vi "IDE_Example_Milan.vi"() -> ()   [LabVIEW 2020]
uses:
  Console XCtrl/Console_Xctrl.xctl
  Server XCtrl/Server.xctl
  ColorText/Code.xctl
panel:
  in  "Clean":bool
  in  "PC Save":bool
  in  "Selection":bool
  in  "PC path":path
  in  "Files":bool
  in  "Server":bool
  in  "Help":bool
  in  "Server":path(xcontrol)=path "/Users/crogers/GitHub/Summer2020/LabVIEWCode/Servers/Jens.vi"
  out "REPL":string(xcontrol)
  in  "Clear":bool
  in  "Save":bool
  in  "Stop":bool
  in  "Run":bool
  in  "Name":string="code.py"
  in  "Code":string(xcontrol)="import os\n\nfor i in range(10):\n     print(i)\n"
  # "¨Processor"
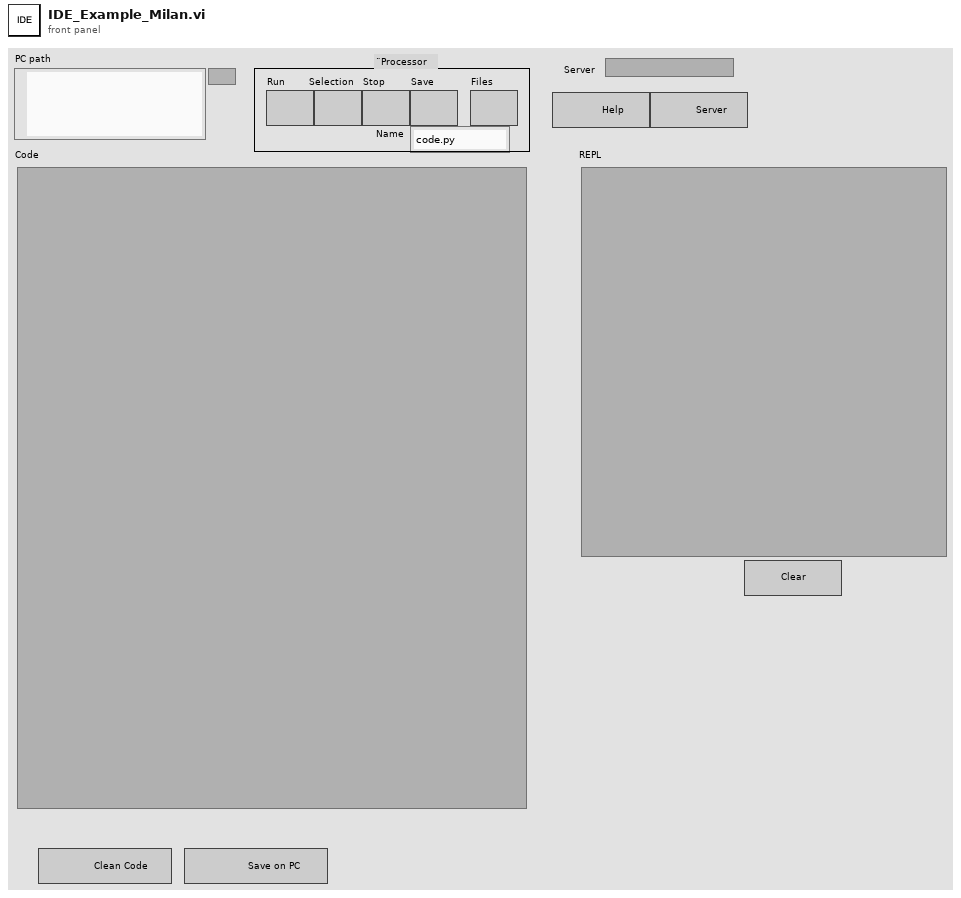
[diagram p1: front panel]
types:
  T1 = cluster{"Quote":u32, "Comment":u32, "Python":u32, "Text":u32, "Triple Quote":u32, "function":u32}
  T2 = enum8{"Enabled", "Disabled", "Disabled and Grayed Out"}
  T3 = typedef "eventvkey.ctl" = enum16{"ASCII", "Enter", "Return", "Shift", "Ctrl", "Alt", "Cmd", "Opt", "Caps", "NumLock", "Clear", "Break", "Up", "Down", "Left", "Right", "Insert", "Delete", "Home", "End", "PageUp", "PageDown", "Escape", "Help", "Pause", "ScrollLock", "F1", "F2", "F3", "F4", "F5", "F6", "F7", "F8", "F9", "F10", "F11", "F12", "F13", "F14", "F15", "F16", "F17", "F18", "F19", "F20", "F21", "F22", "F23", "F24", "Play", "VolumeUp", "VolumeDown", "Mute", "Two Byte Char"}
  T4 = cluster{"Shift":bool, "Ctrl":bool, "Alt":bool, "Cmd":bool, "Opt":bool}
  T5 = cluster{"Char":i16, "VKey":T3, "PlatMods":cluster{"Shift":bool, "Ctrl":bool, "Alt":bool, "Cmd":bool, "Opt":bool}}
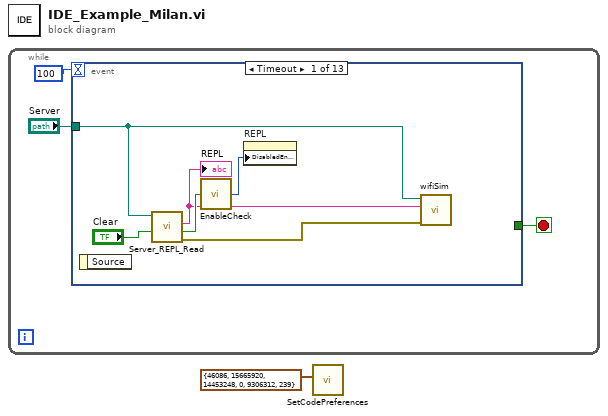
[diagram p0: block diagram]
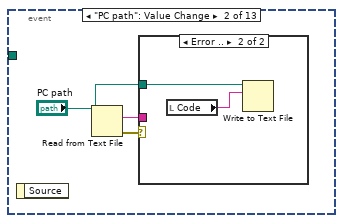
[diagram p2: hidden frame]
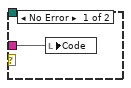
[diagram p3: hidden frame]
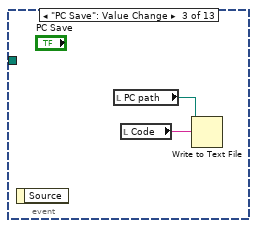
[diagram p4: hidden frame]
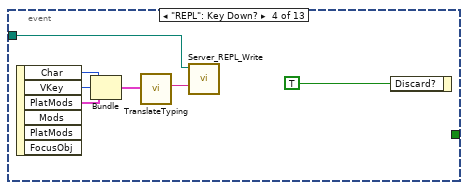
[diagram p5: hidden frame]
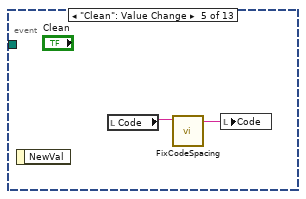
[diagram p6: hidden frame]
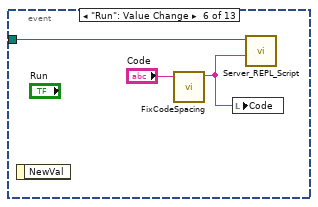
[diagram p7: hidden frame]
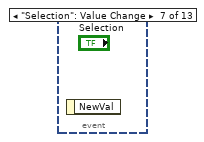
[diagram p8: hidden frame]
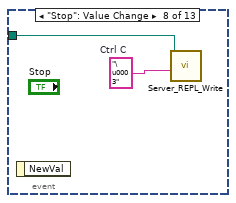
[diagram p9: hidden frame]
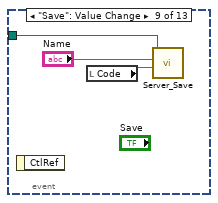
[diagram p10: hidden frame]
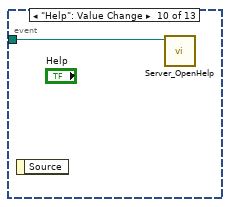
[diagram p11: hidden frame]
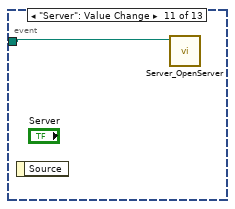
[diagram p12: hidden frame]
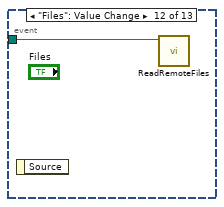
[diagram p13: hidden frame]
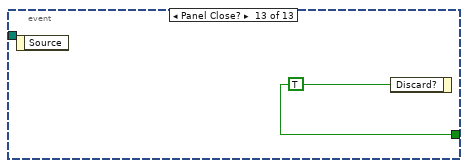
[diagram p14: hidden frame]
diagram:
  n1 = while {
    stop <- w3 stop-if-true
    n2 = event shown="[0] Timeout" {
      selector: _ -> [_ _ _ _ _ _ _ _ _ _ _ _ _]
      dyn-events: _ -> [_ _ _ _ _ _ _ _ _ _ _ _ _]
      timeout: 100 -> [_ _ _ _ _ _ _ _ _ _ _ _ _]
      tunnel: [_ _ _ _ _ _ _ _ _ _ _ _ w39] -> w3
      tunnel: "Server" -> [w5 _ _ w19 _ w29 _ w31 w33 w36 w37 w38 _]
      event Timeout {
        n3 = event-data() -> ()  [unwired: 1 in, 1 out]
        n4 = call "Server_REPL_Read.vi"("Clear"="Clear", "Server"=w5) -> ("error out"=w6:errorcluster, "Running?"=w9:bool, "REPL"=w7:string)  [unwired: 7 in]
        "REPL" <- w7
        n5 = call "EnableCheck.vi"("Enable?"=w9) -> ("Enum"=w10:T2)
        n6 = property on="REPL" class="Console_Xctrl (strict)"("DisabledEnum"=w10) -> ()  [unwired: 2 in, 2 out]
        n7 = call "wifiSim.vi"("error in (no error)"=w6, "REPL"=w7, "Server"=w5) -> ()  [unwired: 9 in]
      }
      event "PC path": Value Change {
        n8 = event-data() -> ()  [unwired: 1 in, 1 out]
        n9 = Read from Text File(file (use dialog)="PC path") -> (text=w12:string, error out=w13:errorcluster)  [unwired: 3 in, 2 out]
        n10 = case shown="Error .." w13 {
          tunnel: w12 -> [w14 _]
          tunnel: "PC path" -> [_ w16]
          frame No Error {
            n11 = local write "Code"(w14) -> ()
          }
          frame Error {
            n12 = local read "Code"() -> (w15:string)
            n13 = Write to Text File(file (use dialog)=w16, text=w15) -> ()  [unwired: 2 in, 3 out]
          }
        }
      }
      event "PC Save": Value Change {
        n14 = event-data() -> ()  [unwired: 1 in, 1 out]
        n15 = local read "PC path"() -> (w18:path)
        n16 = local read "Code"() -> (w17:string)
        n17 = Write to Text File(file (use dialog)=w18, text=w17) -> ()  [unwired: 2 in, 3 out]
      }
      event "REPL": Key Down? {
        n18 = event-data() -> ("Char"=w24:i16, "VKey"=w23:T3, "PlatMods"=w21:T4)  [unwired: 1 in, 3 out]
        n19 = Bundle("Char"=w24, "VKey"=w23, "PlatMods"=w21) -> (w25:T5)  [unwired: 1 in]
        n20 = call "TranslateTyping.vi"("Cluster"=w25) -> ("key"=w20:string)  [unwired: 10 in]
        n21 = call "Server_REPL_Write.vi"("Code"=w20, "Server"=w19) -> ()  [unwired: 9 in, 1 out]
        n22 = event-data("Discard?"=TRUE) -> ()  [unwired: 1 in, 1 out]
      }
      event "Clean": Value Change {
        n23 = event-data() -> ()  [unwired: 1 in, 1 out]
        n24 = local read "Code"() -> (w26:string)
        n25 = call "FixCodeSpacing.vi"("Code"=w26) -> ("Cleaned"=w27:string)  [unwired: 10 in]
        n26 = local write "Code"(w27) -> ()
      }
      event "Run": Value Change {
        n27 = event-data() -> ()  [unwired: 1 in, 1 out]
        n28 = call "FixCodeSpacing.vi"("Code"="Code") -> ("Cleaned"=w28:string)  [unwired: 10 in]
        n29 = local write "Code"(w28) -> ()
        n30 = call "Server_REPL_Script.vi"("Code"=w28, "Server"=w29) -> ()  [unwired: 9 in, 1 out]
      }
      event "Selection": Value Change {
        n31 = event-data() -> ()  [unwired: 1 in, 1 out]
      }
      event "Stop": Value Change {
        w32 = "\u0003"  # Ctrl C
        n32 = event-data() -> ()  [unwired: 1 in, 1 out]
        n33 = call "Server_REPL_Write.vi"("Code"=w32, "Server"=w31) -> ()  [unwired: 9 in, 1 out]
      }
      event "Save": Value Change {
        n34 = event-data() -> ()  [unwired: 1 in, 1 out]
        n35 = local read "Code"() -> (w35:string)
        n36 = call "Server_Save.vi"("Code"=w35, "Name"="Name", "Server"=w33) -> ()  [unwired: 8 in, 1 out]
      }
      event "Help": Value Change {
        n37 = event-data() -> ()  [unwired: 1 in, 1 out]
        n38 = call "Server_OpenHelp.vi"("Server"=w36) -> ()  [unwired: 10 in, 1 out]
      }
      event "Server": Value Change {
        n39 = event-data() -> ()  [unwired: 1 in, 1 out]
        n40 = call "Server_OpenServer.vi"("Server"=w37) -> ()  [unwired: 10 in, 1 out]
      }
      event "Files": Value Change {
        n41 = event-data() -> ()  [unwired: 1 in, 1 out]
        n42 = call "ReadRemoteFiles.vi"("Server"=w38) -> ()  [unwired: 11 in]
      }
      event Panel Close? {
        w39 = TRUE ("Discard?")
        n43 = event-data() -> ()  [unwired: 1 in, 1 out]
        n44 = event-data("Discard?"=w39) -> ()  [unwired: 1 in, 1 out]
      }
    }
  }
  n45 = call "SetCodePreferences.vi"("Color choices"=T1 {"Quote"=46086, "Comment"=15665920, "Python"=14453248, "Text"=0, "Triple Quote"=9306312, "function"=239}) -> ()  [unwired: 11 in]
